vi "Get Source Inclusion.vi"(8 "error IO":errorcluster, 10 "Item ID":string, 11 "sourceItems":refnum<class "AB_Source.lvclass">[](array[class])) -> (0 "error out":errorcluster, 3 "sourceInclusion":T1)   [LabVIEW 2020, in "NI_AB_API_PPL.lvclass"]
uses:
  <vilib>/AppBuilder/AB_API/PPL/NI_AB_API_PPL.lvclass
  <vilib>/AppBuilder/AB_Source_Inclusion.ctl
  <vilib>/AppBuilder/AB_Classes/Source/AB_Source.lvclass
  <vilib>/AppBuilder/AB_API/PPL/NI_AB_API_PPL.lvclass/NI_AB_API_PPL.ctl
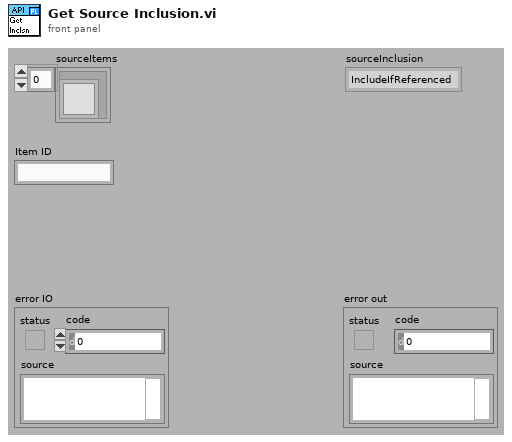
[diagram p1: front panel]
types:
  T1 = typedef "AB_Source_Inclusion.ctl" = enum16{"IncludeIfReferenced", "Include", "Exclude", "TopLevel"}
  T2 = typedef "AB_Source.ctl" = cluster{"path":path, "itemID":string, "parentIndex":i32, "sourceInclusion":T1, "destinationIndex":i32, "properties":T3[], "newName":string, "lvfile":bool, "valid":bool, "eng_inBuild":bool, "eng_isNonVILink":bool, "Amalgamation":bool, "Amalgamation Piece":bool, "eng_delimitedName":string, "preventRename":bool}
  T3 = typedef "AB_Source_Properties.ctl" = cluster{"sourcePropertyType":T4, "value":variant}
  T4 = typedef "AB_Source_Property_Type.ctl" = enum16{"Remove block diagram", "Remove front panel", "Password", "Window has title bar", "Show menu bar", "Show vertical scroll bar", "Show horizontal scroll bar", "Show toolbar", "Show Abort button", "Show fp when called", "Window behavior", "Allow user to close window", "Window run-time position", "Run when opened", "Allow debugging", "Auto error handling", "Generate guard code", "Use stack variables", "Expression folding", "Integer only", "Inline subVI"}
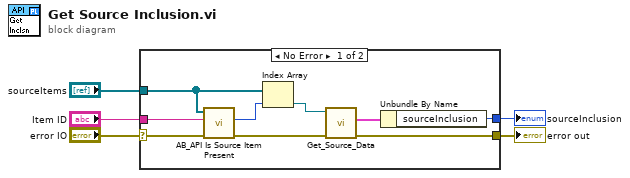
[diagram p0: block diagram]
diagram:
  n1 = case shown="No Error" "error IO" {
    selector: "error IO" -> [w6 w15]
    tunnel: [w14 _] -> w5
    tunnel: [w12 w15] -> w4
    tunnel: "sourceItems" -> [w8 _]
    tunnel: "Item ID" -> [w7 _]
    frame No Error {
      n2 = call <vilib>:"AB_API Is Source Item Present.vi"("error in"=w6, "item ID"=w7, "source items"=w8) -> ("error out"=w11:errorcluster, "index"=w10:i32)  [unwired: 7 out]
      n3 = Index Array(array=w8, index=w10) -> (element=w9:refnum<class "AB_Source.lvclass">)
      n4 = call <vilib>:"Get_Source_Data.vi"("error in (no error)"=w11, "Class in"=w9) -> ("error out"=w12:errorcluster, "data"=w13:T2)  [unwired: 7 in, 1 out]
      n5 = Unbundle By Name(w13) -> ("sourceInclusion"=w14:T1)
    }
    frame Error {
    }
  }
  "sourceInclusion" <- w5
  "error out" <- w4
